vi "low priority dash data.vi"() -> ()   [LabVIEW 2012]
panel:
  in  "String":string
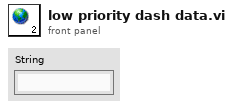
[diagram p1: front panel]
diagram:
